vi "updateDataOut.vi"(8 "error in (no error)":errorcluster) -> (0 "error out":errorcluster)   [LabVIEW 2017]
uses:
  TypeDefs/UDPListenFGVCtrl.ctl
  TypeDefs/dataOut.ctl
  TypeDefs/dataFGVState.ctl
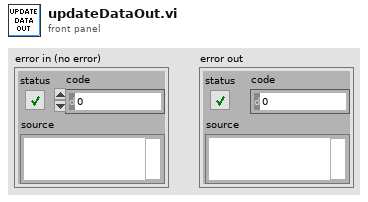
[diagram p1: front panel]
types:
  T1 = typedef "dataFGVState.ctl" = enum16{"init", "write data out", "read data out", "write data in", "read data in"}
  T2 = typedef "UDPListenFGVCtrl.ctl" = enum16{"Read", "Write"}
  T3 = typedef "dataOut.ctl" = cluster{"X0pos":dbl, "Y0pos":dbl, "Z0pos":dbl, "Fx":dbl, "Fy":dbl, "Fz":dbl, "Encoder1":i32, "Encoder2":i32, "Pot1":dbl, "Pot2":dbl, "Theta0":dbl, "Theta1":dbl, "X1pos":dbl, "Y1pos":dbl, "Z1pos":dbl, "X2pos":dbl, "Y2pos":dbl, "Z2pos":dbl, "ErrorOccurred":bool}
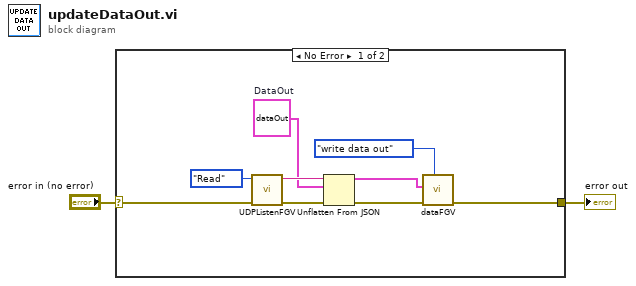
[diagram p0: block diagram]
diagram:
  n1 = case shown="No Error" "error in (no error)" {
    selector: "error in (no error)" -> [w4 w12]
    tunnel: [w3 w12] -> w1
    frame No Error {
      w9 = T3 {"X0pos"=0.0, "Y0pos"=0.0, "Z0pos"=0.0, "Fx"=0.0, "Fy"=0.0, "Fz"=0.0, "Encoder1"=0, "Encoder2"=0, "Pot1"=0.0, "Pot2"=0.0, "Theta0"=0.0, "Theta1"=0.0, "X1pos"=0.0, "Y1pos"=0.0, "Z1pos"=0.0, "X2pos"=0.0, "Y2pos"=0.0, "Z2pos"=0.0, "ErrorOccurred"=FALSE}  # DataOut
      n2 = call "UDPListenFGV.vi"("error in (no error)"=w4, "Enum"=UDPListenFGVCtrl."Read") -> ("error out"=w8:errorcluster, "Read Data"=w10:string)  [unwired: 8 in]
      n3 = Unflatten From JSON(JSON string=w10, type and defaults=w9, error in (no error)=w8) -> (value=w7:T3, error out=w5:errorcluster)  [unwired: 4 in]
      n4 = call "dataFGV.vi"("Enum"=dataFGVState."write data out", "error in (no error)"=w5, "DataOut"=w7) -> ("error out"=w3:errorcluster)  [unwired: 6 in, 2 out]
    }
    frame Error {
    }
  }
  "error out" <- w1
